vi "Add_Result_OPC_Fixture.vi"(3 "Number Product":i32, 4 "Condition Test":string(combo)="D_L", 5 "Fixture Data input":u16[](array[numeric])) -> (2 "Fixture Data output":u16[](array[numeric]))   [LabVIEW 2017]
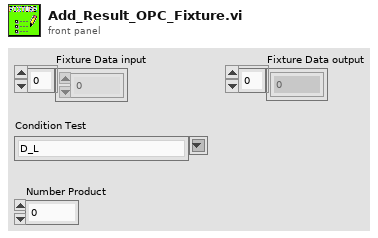
[diagram p1: front panel]
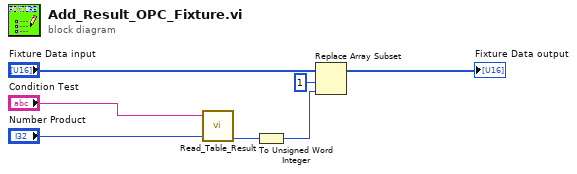
[diagram p0: block diagram]
diagram:
  n1 = call "Read_Table_Result.vi"("Condition Test"="Condition Test", "Number Product"="Number Product") -> ("Num Result"=w2:u8)  [unwired: 3 in, 5 out]
  n2 = To Unsigned Word Integer(number=w2) -> (unsigned 16bit integer=w1:u16)
  n3 = Replace Array Subset(array="Fixture Data input", new element=w1, index=1) -> (→"Fixture Data output":u16[])
